vi "searchAndGetIndex.vi"() -> ()   [LabVIEW 2017]
panel:
  out "indexsWhereTrue":i32[](array[numeric])
  in  "lessThan":i32=13
  out "x < y?":bool[](array[boolean])
  out "Array":i32[](array[numeric])
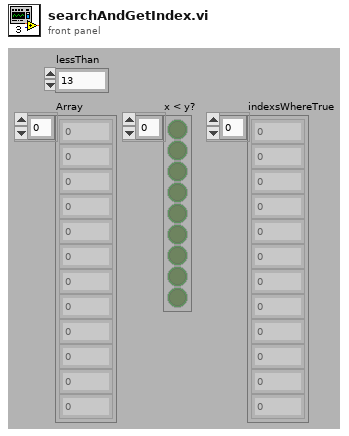
[diagram p1: front panel]
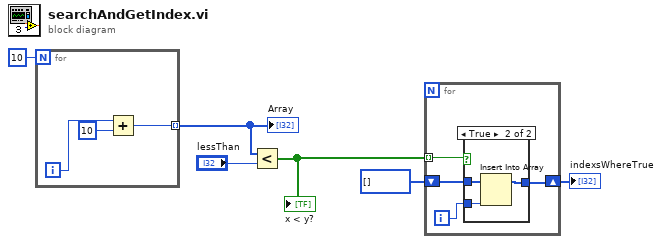
[diagram p0: block diagram]
diagram:
  n1 = for {
    N: 10 -> [_]
    tunnel: [w7] -> w5 mode=indexing
    i -> [w9]
    n2 = Add(x=w9, y=10) -> (x+y=w7:i32)
  }
  "Array" <- w5
  n3 = Less?(x=w5, y="lessThan") -> (x < y?=w3:bool[])
  "x < y?" <- w3
  n4 = for {
    tunnel: w3 -> [w13] mode=indexing
    shift-right: [w10] -> w1
    shift-left: i32[] [] -> [w11]
    i -> [w12]
    n5 = case shown="True" w13 {
      tunnel: w12 -> [_ w16]
      tunnel: w11 -> [w14 w17]
      tunnel: [w14 w15] -> w10
      frame False {
      }
      frame True {
        n6 = Insert Into Array(array=w17, new element=w16) -> (w15:i32[])  [unwired: 1 in]
      }
    }
  }
  "indexsWhereTrue" <- w1
